vi "Config Instrument.vi"(0 "VISA resource name":refnum<visa-resource-name>, 1 "Monitor Output (7: VMIX)":u16(ring)=7 items=["Off", "CS NEG", "CS POS", "VAD", "VCM NEG", "VCM POS", "VDIF", "VMIX"], 5 "Excitation Frequency (1: 13.7 Hz)":u16(ring)=1 items=["9.8 Hz", "13.7 Hz", "16.2 Hz"], 7 "CMR (T: On)":bool=TRUE, 9 "Guard Drive (F: Off)":bool, 11 "error in (no error)":errorcluster, 12 "Change All or One (0: Change One)":u16(ring) items=["Change One", "Change All"]) -> (4 "VISA resource name out":refnum<visa-resource-name>, 15 "error out":errorcluster)   [LabVIEW 2019, in "Lake Shore Cryotronics 370.lvlib"]
doc: "This VI configures the instrument set up. Parameters configured are;\nExcitation Frequency, Common Mode Reduction, Guard Drive, Monitor Output, Change All or One."
uses:
  Lake Shore Cryotronics 370.lvlib
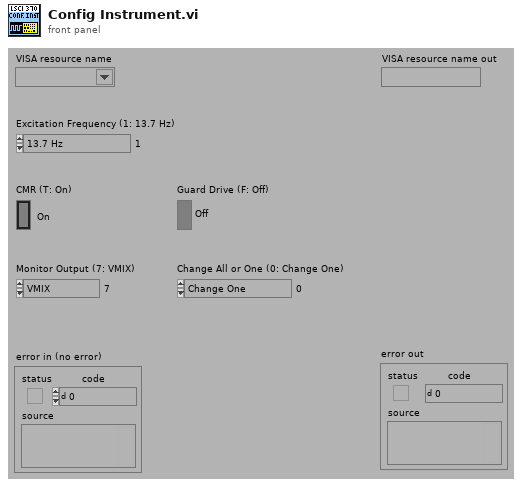
[diagram p1: front panel]
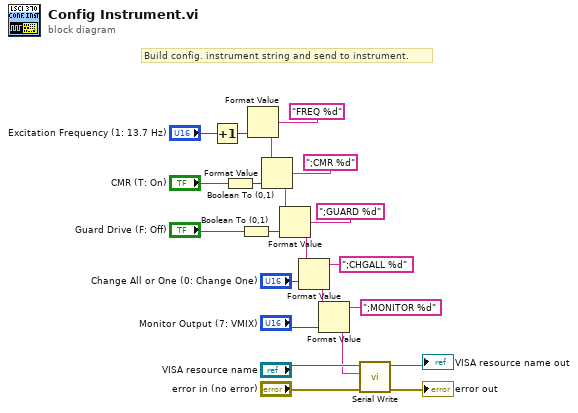
[diagram p0: block diagram]
diagram:
  # "Build config. instrument string and send to instrument."
  n1 = Increment(x="Excitation Frequency (1: 13.7 Hz)") -> (x+1=w11:u16)
  n2 = Boolean To (0,1)(Boolean="CMR (T: On)") -> (0, 1=w9:i16)
  n3 = Boolean To (0,1)(Boolean="Guard Drive (F: Off)") -> (0, 1=w6:i16)
  n4 = Format Value(format string="FREQ %d", value (0)=w11) -> (output string=w19:string)  [unwired: 1 in]
  n5 = Format Value(string ("")=w19, format string=";CMR %d", value (0)=w9) -> (output string=w13:string)
  n6 = Format Value(string ("")=w13, format string=";GUARD %d", value (0)=w6) -> (output string=w12:string)
  n7 = Format Value(string ("")=w12, format string=";CHGALL %d", value (0)="Change All or One (0: Change One)") -> (output string=w3:string)
  n8 = Format Value(string ("")=w3, format string=";MONITOR %d", value (0)="Monitor Output (7: VMIX)") -> (output string=w1:string)
  n9 = call "Serial Write.vi"("error in (no error)"="error in (no error)", "Write Buffer (\"\")"=w1, "VISA resource name"="VISA resource name") -> ("error out"=→"error out":errorcluster, "VISA resource name out"=→"VISA resource name out":refnum<visa-resource-name>)  [unwired: 6 in, 1 out]
